vi "HB_ConfigureLED.vi"(0 "HBDevRef":T2, 5 "LED Strip Channel":T1=enum."HB GPIO 0", 7 "LED Model":enum8{"WS2812", "WS2812B"}(ring), 9 "Number of LEDs":u8=1 min=1 step=1, 11 "error in (no error)":errorcluster) -> (4 "HBDevRef":T2, 15 "error out":errorcluster)   [LabVIEW 2018]
doc: "Configures the specified DIO channel to drive an LED strip with the specified number of LEDs. The LED Model control specifies the LED strip models that are supported by the Huskie Board. The Huskie Board can only drive a single LED strip. Configuring subsequent LEDs, unconfigures previously configured LEDs."
uses:
  <vilib>/Rock Robotics/WPI/SerialPort/WPI_SerialPortRef.ctl
  LED Channels.ctl
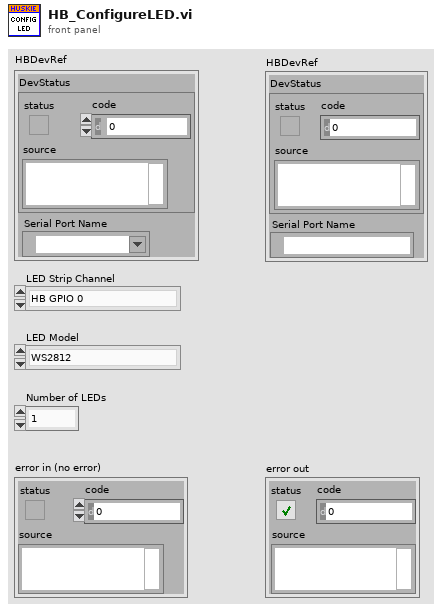
[diagram p1: front panel]
types:
  T1 = typedef "LED Channels.ctl" = enum8{"SD card D1", "SD card D0", "SD card CLK", "SD card CMD", "SD card D2", "SD card D3", "roboRIO MOSI", "roboRIO MISO", "roboRIO CLK", "roboRIO CS", "roboRIO UART RX", "roboRIO UART TX", "roboRIO SCL", "robotRIO SDA", "HB GPIO 0", "HB GPIO 1", "HB GPIO 2", "HB GPIO 3", "HB LCD", "ADC CS2", "ADC CS1", "ADC DO", "ADC CLK", "ADC DI", "LED 1", "LED 2", "LED 3", "LED 4", "EEPROM SCL", "EEPROM SDA", "USB UART TX", "USB UART RX"}
  T2 = typedef "WPI_SerialPortRef.ctl" = cluster{"DevStatus":errorcluster, "Serial Port Name":refnum<visa-resource-name>}
  T3 = enum8{"SD card D1", "SD card D0", "SD card CLK", "SD card CMD", "SD card D2", "SD card D3", "roboRIO MOSI", "roboRIO MISO", "roboRIO CLK", "roboRIO CS", "roboRIO UART RX", "roboRIO UART TX", "roboRIO SCL", "robotRIO SDA", "HB GPIO 0", "HB GPIO 1", "HB GPIO 2", "HB GPIO 3", "HB LCD", "ADC CS2", "ADC CS1", "ADC DO", "ADC CLK", "ADC DI", "LED 1", "LED 2", "LED 3", "LED 4", "EEPROM SCL", "EEPROM SDA", "USB UART TX", "USB UART RX"}[]
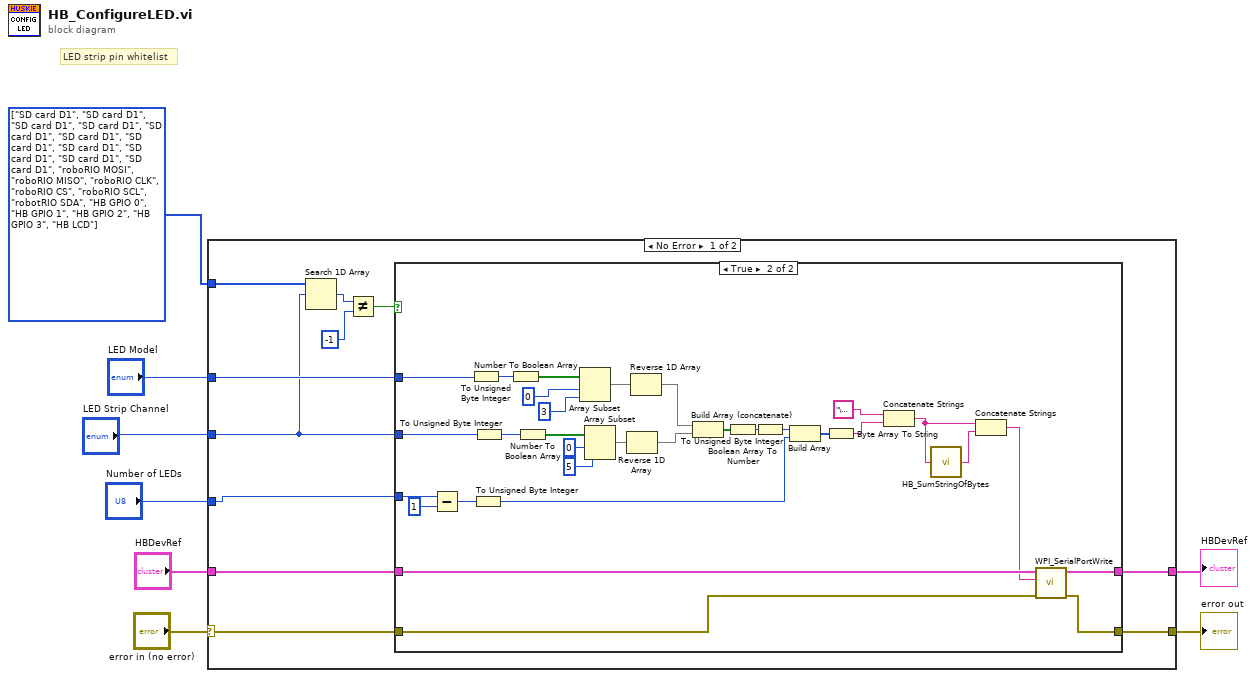
[diagram p0: block diagram]
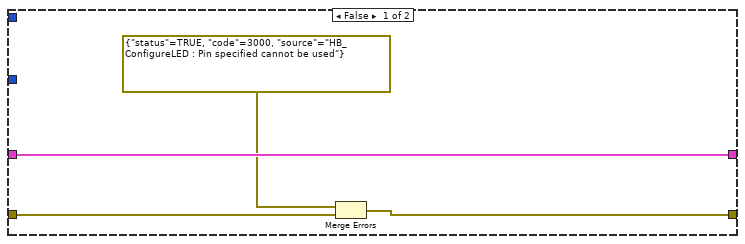
[diagram p2: hidden frame]
diagram:
  w2 = T3 [enum."SD card D1", enum."SD card D1", enum."SD card D1", enum."SD card D1", enum."SD card D1", enum."SD card D1", enum."SD card D1", enum."SD card D1", enum."SD card D1", enum."SD card D1", enum."SD card D1", enum."roboRIO MOSI", enum."roboRIO MISO", enum."roboRIO CLK", enum."roboRIO CS", enum."roboRIO SCL", enum."robotRIO SDA", enum."HB GPIO 0", enum."HB GPIO 1", enum."HB GPIO 2", enum."HB GPIO 3", enum."HB LCD"] items=["SD card D1", "SD card D0", "SD card CLK", "SD card CMD", "SD card D2", "SD card D3", "roboRIO MOSI", "roboRIO MISO", "roboRIO CLK", "roboRIO CS", "roboRIO UART RX", "roboRIO UART TX", "roboRIO SCL", "robotRIO SDA", "HB GPIO 0", "HB GPIO 1", "HB GPIO 2", "HB GPIO 3", "HB LCD", "ADC CS2", "ADC CS1", "ADC DO", "ADC CLK", "ADC DI", "LED 1", "LED 2", "LED 3", "LED 4", "EEPROM SCL", "EEPROM SDA", "USB UART TX", "USB UART RX"]
  # "LED strip pin whitelist"
  n1 = case shown="No Error" "error in (no error)" {
    selector: "error in (no error)" -> [w16 w55]
    tunnel: "HBDevRef" -> [w19 w56]
    tunnel: [w18 w55] -> w7
    tunnel: [w17 w56] -> w6
    tunnel: "LED Strip Channel" -> [w11 _]
    tunnel: "LED Model" -> [w15 _]
    tunnel: "Number of LEDs" -> [w14 _]
    tunnel: w2 -> [w10 _]
    frame No Error {
      n2 = Search 1D Array(1D array=w10, element=w11) -> (index of element=w13:i32)  [unwired: 1 in]
      n3 = Not Equal?(x=w13, y=-1) -> (x != y?=w9:bool)
      n4 = case shown="True" w9 {
        tunnel: w19 -> [w23 w54]
        tunnel: [w21 w53] -> w18
        tunnel: [w23 w52] -> w17
        tunnel: w16 -> [w22 w42]
        tunnel: w15 -> [_ w41]
        tunnel: w14 -> [_ w26]
        tunnel: w11 -> [_ w24]
        frame False {
          n5 = Merge Errors(errorcluster {"status"=TRUE, "code"=3000, "source"="HB_ConfigureLED : Pin specified cannot be used"} ("error in"), w22) -> (w21:errorcluster)
        }
        frame True {
          n6 = Subtract(x=w26, y=u8 1) -> (x-y=w27:u8)
          n7 = To Unsigned Byte Integer(number=w41) -> (unsigned 8bit integer=w40:u8)
          n8 = To Unsigned Byte Integer(number=w27) -> (unsigned 8bit integer=w29:u8)
          n9 = To Unsigned Byte Integer(number=w24) -> (unsigned 8bit integer=w47:u8)
          n10 = Number To Boolean Array(number=w40) -> (Boolean array=w39:bool[])
          n11 = Number To Boolean Array(number=w47) -> (Boolean array=w43:bool[])
          n12 = Array Subset(array=w39, index=0, length=3) -> (w30:bool[])
          n13 = Array Subset(array=w43, index=0, length=5) -> (w44:bool[])
          n14 = Reverse 1D Array(array=w44) -> (reversed array=w34:bool[])
          n15 = Reverse 1D Array(array=w30) -> (reversed array=w28:bool[])
          n16 = Build Array (concatenate)(w28, w34) -> (w33:bool[])
          n17 = Boolean Array To Number(Boolean array=w33) -> (number=w37:u32)
          n18 = To Unsigned Byte Integer(number=w37) -> (unsigned 8bit integer=w36:u8)
          n19 = Build Array(w36, w29) -> (w35:u8[])
          n20 = Byte Array To String(unsigned byte array=w35) -> (string=w32:string)
          n21 = Concatenate Strings("\u0017", w32) -> (w49:string)
          n22 = call <vilib>:"HB_SumStringOfBytes.vi"("String Of Bytes"=w49) -> ("Sum as String"=w48:string)
          n23 = Concatenate Strings(w49, w48) -> (w50:string)
          n24 = call <vilib>:"WPI_SerialPortWrite.vi"("error in (no error)"=w42, "Buffer"=w50, "SerialPortRef"=w54) -> ("error out"=w53:errorcluster, "SerialPortRef"=w52:T2)  [unwired: 6 in, 1 out]
        }
      }
    }
    frame Error {
    }
  }
  "error out" <- w7
  "HBDevRef" <- w6
